vi "nirviRandomDataMultiElementFPGAFIFO.vi"(0 "Method":T1, 1 "Fifo":T2={"displayName"="", "hardwareName"="", "dataType"=enum."I16", "elementTypeDescriptor"=variant, "terminalTypeDescriptor"=variant, "requestedNumberOfElements"=2, "memoryType"=enum."Look-Up Table", "arbitrationForInterfaceA"=enum."Arbitrate if Multiple Requestors Only", "numberOfElementsPerRead"=1, "arbitrationForInterfaceB"=enum."Always Arbitrate", "numberOfElementsPerWrite"=1, "VI_Defined"=FALSE, "type"=enum."Target-Scoped", "initializationParameters"={"initialized"=FALSE, "VI_Path"=path "", "initialData"=variant}, "disableOnOverflow/Underflow"=FALSE, "interfaceConfiguration"=enum."Read A-Write B", "controlLogic"=enum."Slice Fabric", "actualNumberOfElements"=1027, "dramSelection"="", "dramMaxOustandingRequests"=0, "dramIncludeByteEnables"=FALSE, "dramGrantTime"=0, "fullEmulation"=FALSE, "memoryInMultipleClockDomains"=FALSE, "memoryLatency"=1} {"memoryLatency" items=["0", "1", "2", "3"]}, 3 "element in":variant, 5 "error in (no error)":errorcluster, 7 "Element Datatype":i32, 8 "In SCTL":bool, 9 "Input Valid?":bool, 11 "Timeout (ms)":i32, 13 "Ready for Output?":bool) -> (14 "element out":variant, 15 "Timed out":bool, 16 "Ready for Input":bool, 17 "count":u32, 18 "Output Valid":bool, 19 "error out":errorcluster)   [LabVIEW 2020]
uses:
  <vilib>/rvi/DataTransferAndStorage/Container/Common/niFpgaContainerState.ctl
  <vilib>/rvi/DataTransferAndStorage/Container/Common/niFpgaDataTypeControl.ctl
  <vilib>/rvi/DataTransferAndStorage/Container/Common/niFpgaContainerImplementationControl.ctl
  <vilib>/rvi/DataTransferAndStorage/Container/Common/niFpgaContainerArbitrationOptionsControl.ctl
  <vilib>/rvi/DataTransferAndStorage/Container/Common/niFpgaTransferTypeControl.ctl
  <vilib>/rvi/DataTransferAndStorage/Container/Common/niFpgaContainerInitializationParameters.ctl
  <vilib>/rvi/Memory/Memory_Types/niFpgaMemoryInterfaceConfiguration.ctl
  <vilib>/rvi/FIFO/Fifo_Types/niFpgaFifoControlLogicControl.ctl
  <vilib>/rvi/DataTransferAndStorage/Container/Common/niFpgaContainerMemoryLatencyControl.ctl
  <vilib>/rvi/DataTransferAndStorage/Container/Common/niFpgaContainerMethod.ctl
  <vilib>/rvi/interface/RandomDataEmulation/nirviQueueStoreOperation.ctl
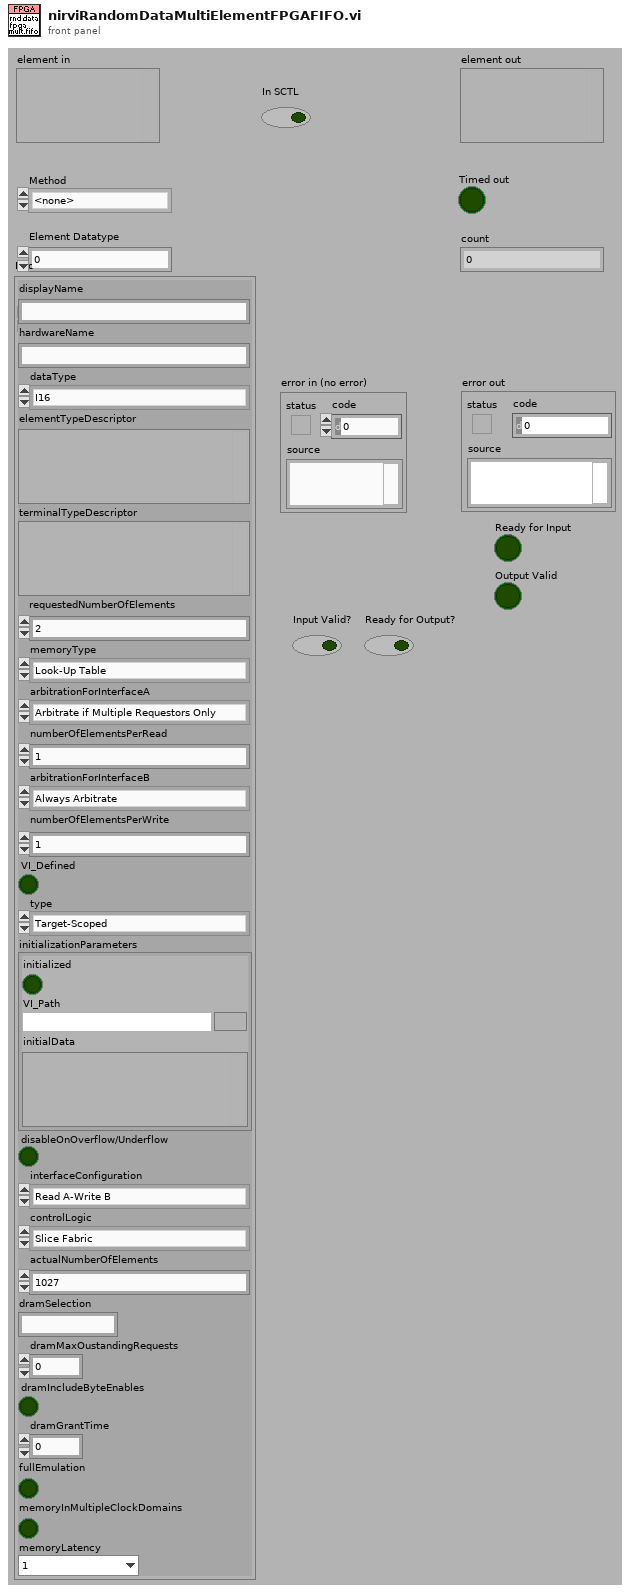
[diagram p1: front panel]
types:
  T1 = typedef "niFpgaContainerMethod.ctl" = enum16{"<none>", "write", "read", "clear", "getNumberOfElementsToWrite", "getNumberOfElementsToRead", "enable", "disable", "flushAndDisable", "getStreamState", "readA", "readB", "dramWrite", "dramWriteWithByteEnables", "dramRequestData", "dramRetrieveData", "readWithoutAcknowledge", "acknowledge", "writeUsingHandshaking", "readUsingHandshaking", "flush"}
  T2 = typedef "niFpgaContainerState.ctl" = cluster{"displayName":string, "hardwareName":string, "dataType":T3, "elementTypeDescriptor":variant, "terminalTypeDescriptor":variant, "requestedNumberOfElements":u32, "memoryType":T4, "arbitrationForInterfaceA":T5, "numberOfElementsPerRead":u32, "arbitrationForInterfaceB":T5, "numberOfElementsPerWrite":u32, "VI_Defined":bool, "type":T6, "initializationParameters":T7, "disableOnOverflow/Underflow":bool, "interfaceConfiguration":T8, "controlLogic":T9, "actualNumberOfElements":u32, "dramSelection":string, "dramMaxOustandingRequests":i32, "dramIncludeByteEnables":bool, "dramGrantTime":u32, "fullEmulation":bool, "memoryInMultipleClockDomains":bool, "memoryLatency":T10}
  T3 = typedef "niFpgaDataTypeControl.ctl" = enum32{"Boolean", "I8", "I16", "I32", "I64", "U8", "U16", "U32", "U64", "FXP", "CustomControl", "SGL"}
  T4 = typedef "niFpgaContainerImplementationControl.ctl" = enum16{"Flip-Flops", "Look-Up Table", "Block Memory", "DRAM", "UltraRAM"}
  T5 = typedef "niFpgaContainerArbitrationOptionsControl.ctl" = enum16{"Always Arbitrate", "Arbitrate if Multiple Requestors Only", "Never Arbitrate"}
  T6 = typedef "niFpgaTransferTypeControl.ctl" = enum16{"Target-Scoped", "Host to Target - DMA", "Target to Host - DMA", "Peer to Peer Reader", "Peer to Peer Writer", "Bidirectional"}
  T7 = typedef "niFpgaContainerInitializationParameters.ctl" = cluster{"initialized":bool, "VI_Path":path, "initialData":variant}
  T8 = typedef "niFpgaMemoryInterfaceConfiguration.ctl" = enum16{"Read A-Write B", "Read A-Read B"}
  T9 = typedef "niFpgaFifoControlLogicControl.ctl" = enum16{"Slice Fabric", "Target Optimal", "Built-in"}
  T10 = typedef "niFpgaContainerMemoryLatencyControl.ctl" = u16
  T11 = typedef "nirviQueueStoreOperation.ctl" = enum16{"Make New Queue", "Get Queue", "Resize Queue", "Close Queues", "Make New Lock", "Get Lock", "Get Host Fifo Size"}
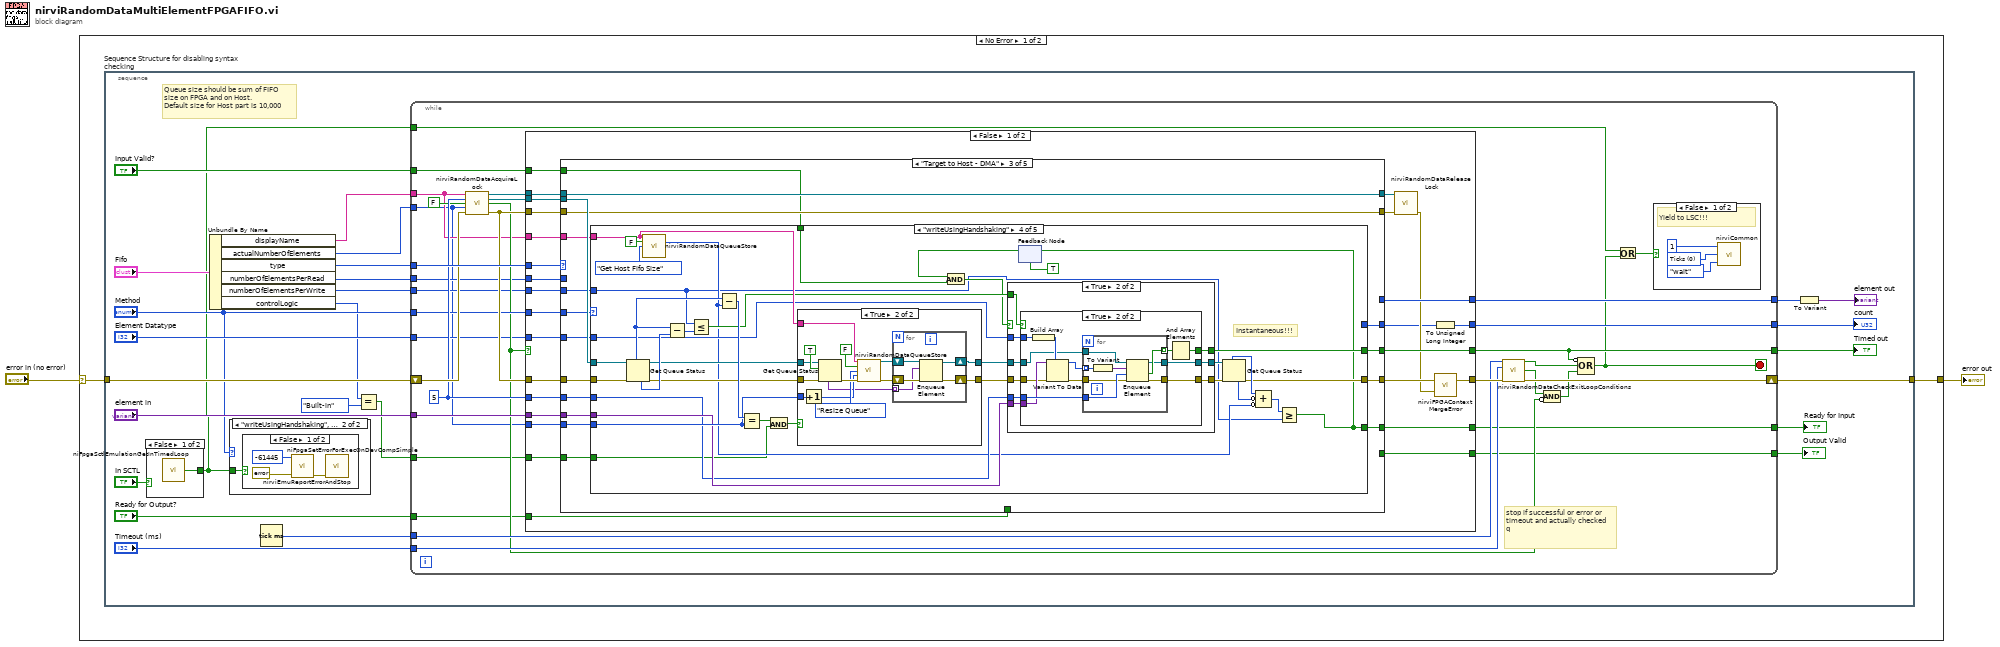
[diagram p0: block diagram]
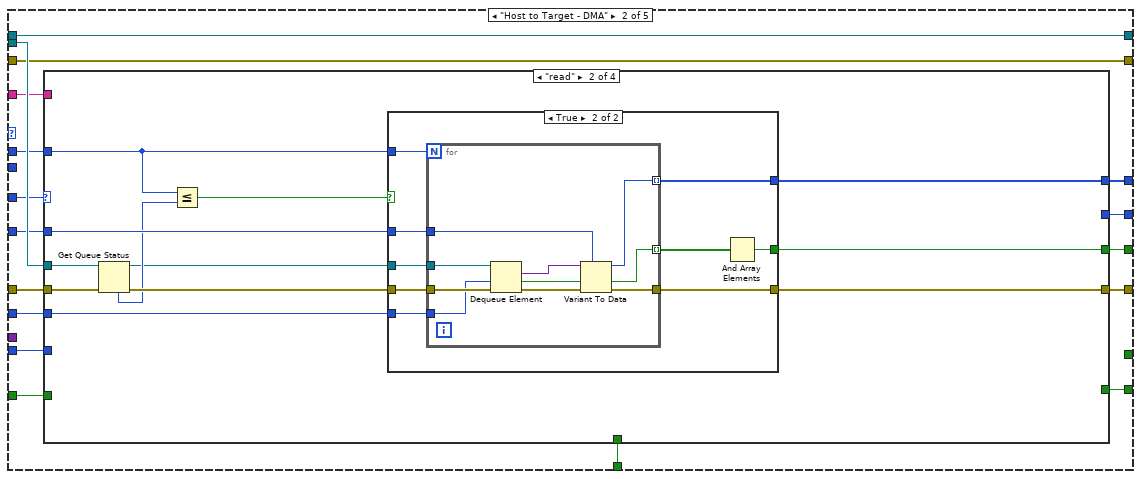
[diagram p7: hidden frame]
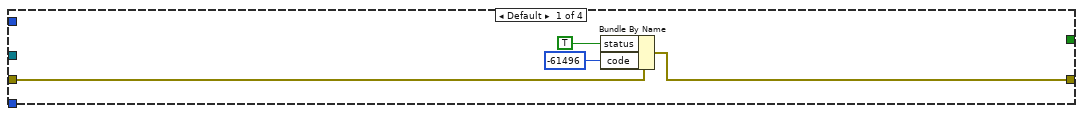
[diagram p8: hidden frame]
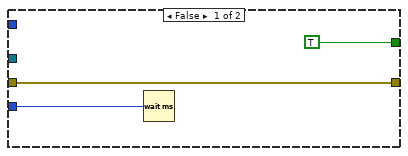
[diagram p9: hidden frame]
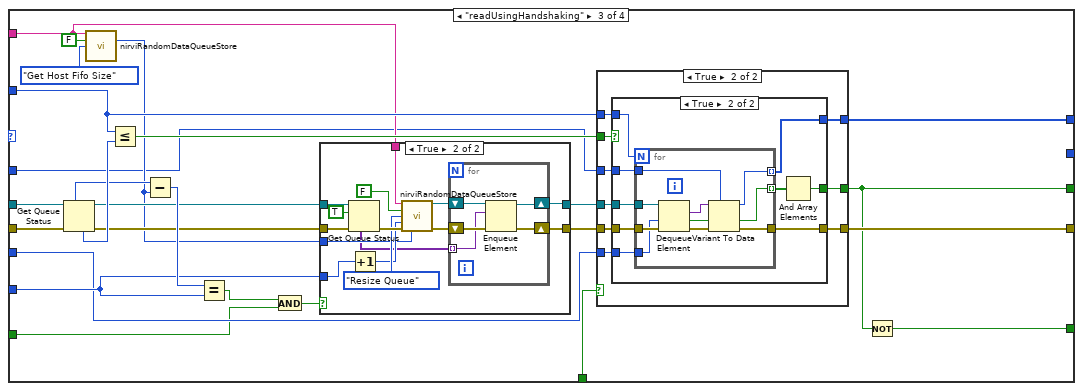
[diagram p10: hidden frame]
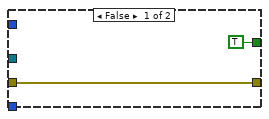
[diagram p11: hidden frame]
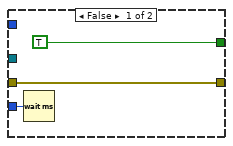
[diagram p12: hidden frame]
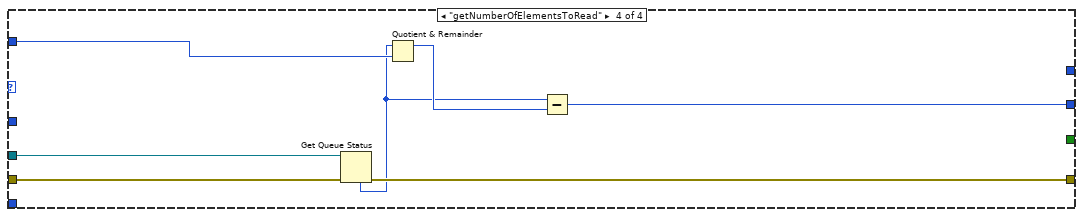
[diagram p14: hidden frame]
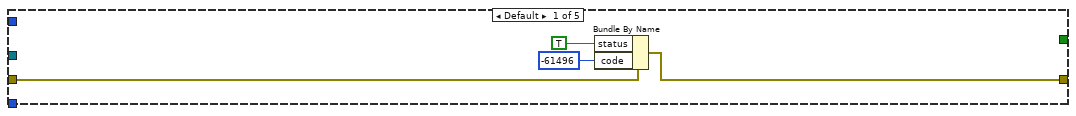
[diagram p15: hidden frame]
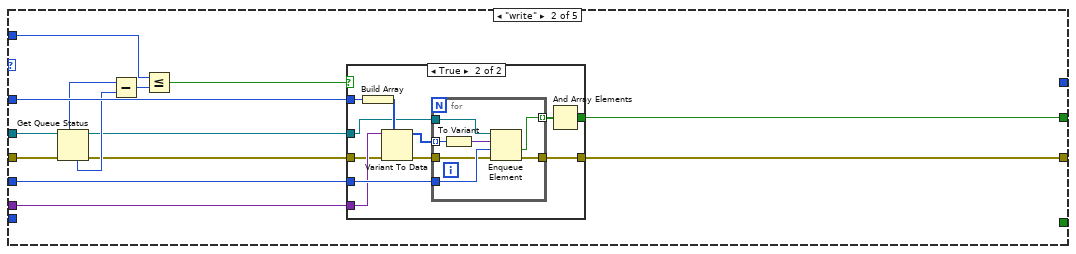
[diagram p16: hidden frame]
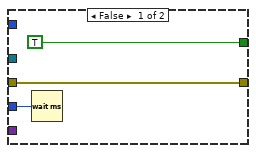
[diagram p17: hidden frame]
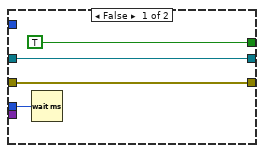
[diagram p20: hidden frame]
diagram:
  n1 = case shown="No Error" "error in (no error)" {
    selector: "error in (no error)" -> [w4 w415]
    tunnel: [w3 w415] -> w2
    frame No Error {
      n2 = stacked-sequence "Sequence Structure for disabling syntax checking" {
        tunnel: w4 -> [w17]
        tunnel: [w29] -> w3
        frame #0 {
          # "Queue size should be sum of FIFO\nsize on FPGA and on Host.\nDefault size for Host part is 10,000"
          n3 = case shown="False" "In SCTL" {
            selector: "In SCTL" -> [_ w32]
            tunnel: [w31 w32] -> w7
            frame False {
              n4 = call <vilib>:"niFpgaSctlEmulationGetInTimedLoop.vi"() -> ("x != 0?"=w31:bool)  [unwired: 15 in]
            }
            frame True {
            }
          }
          n5 = Unbundle By Name("Fifo") -> ("displayName"=w27:string, "actualNumberOfElements"=w25:u32, "type"=w24:T6, "numberOfElementsPerRead"=w20:u32, "numberOfElementsPerWrite"=w19:u32, "controlLogic"=w11:T9)
          n6 = case shown="\"writeUsingHandshaking\", \"readUsingHandshaking\"" "Method" {
            tunnel: w7 -> [_ w33]
            frame Default {
            }
            frame "writeUsingHandshaking", "readUsingHandshaking" {
              n7 = case shown="False" w33 {
                frame False {
                  n8 = call <vilib>:"niFpgaSetErrorForExecOnDevCompSimple.vi"("error code"=-61445, "error in"=errorcluster {"status"=FALSE, "code"=0, "source"=""}) -> ("error out"=w36:errorcluster)  [unwired: 13 in]
                  n9 = call <vilib>:"nirviEmuReportErrorAndStop.vi"("error to report"=w36) -> ()  [unwired: 1 in, 14 out]
                }
                frame True {
                }
              }
            }
          }
          n10 = Tick Count (ms)() -> (millisecond timer value=w28:u32)
          n11 = Equal?(x=w11, y=niFpgaFifoControlLogicControl."Built-in") -> (x = y?=w9:bool)
          n12 = while {
            tunnel: w24 -> [w67]
            tunnel: "element in" -> [w69]
            tunnel: "Timeout (ms)" -> [w63]
            tunnel: [w68] -> w6
            tunnel: [w55] -> w22
            tunnel: w28 -> [w64]
            tunnel: w27 -> [w46]
            shift-right: [w66] -> w29
            shift-left: w17 -> [w62]
            tunnel: w25 -> [w45]
            tunnel: "Method" -> [w56]
            tunnel: [w54] -> w21
            tunnel: "Element Datatype" -> [w49]
            tunnel: w20 -> [w48]
            tunnel: w19 -> [w47]
            tunnel: "Ready for Output?" -> [w44]
            tunnel: [w43] -> w14
            tunnel: "Input Valid?" -> [w42]
            tunnel: [w41] -> w12
            tunnel: w9 -> [w40]
            tunnel: w7 -> [w38]
            stop <- w39 stop-if-true
            w60 = 5 ("ms timeout (-1)")
            # "stop if successful or error or \ntimeout and actually checked q"
            n13 = call <vilib>:"nirviRandomDataAcquireLock.vi"("name"=w46, "ms timeout (-1)"=w60, "Host?"=FALSE, "fpga fifo size"=w45, "error in (no error)"=w62) -> ("lock out"=w61:refnum<queue>, "queue out"=w58:refnum<queue>, "timed out"=w53:bool, "error out"=w57:errorcluster)  [unwired: 7 out]
            n14 = case shown="False" w53 {
              selector: w53 -> [_ w414]
              tunnel: w69 -> [w85 _]
              tunnel: w60 -> [w99 _]
              tunnel: [w98 _] -> w68
              tunnel: [w94 w413] -> w65
              tunnel: [w97 w414] -> w55
              tunnel: w67 -> [w96 _]
              tunnel: w57 -> [w91 w413]
              tunnel: w61 -> [w86 _]
              tunnel: w58 -> [w92 _]
              tunnel: w57 -> [w89 _]
              tunnel: w56 -> [w88 _]
              tunnel: [w83 _] -> w54
              tunnel: w49 -> [w82 _]
              tunnel: w48 -> [w81 _]
              tunnel: w47 -> [w80 _]
              tunnel: w46 -> [w79 _]
              tunnel: w45 -> [w78 _]
              tunnel: w44 -> [w77 _]
              tunnel: [w76 _] -> w43
              tunnel: w42 -> [w75 _]
              tunnel: [w74 _] -> w41
              tunnel: w40 -> [w73 _]
              frame False {
                n15 = case shown="\"Target to Host - DMA\"" w96 {
                  tunnel: w99 -> [_ w118 w259 _ _]
                  tunnel: [_ w117 w257 _ _] -> w97
                  tunnel: [w102 w119 w260 w406 w407] -> w95
                  tunnel: [_ w109 _ _ _] -> w98
                  tunnel: w85 -> [_ _ w258 _ _]
                  tunnel: w91 -> [w102 w116 w256 w406 w408]
                  tunnel: w92 -> [_ w115 w255 _ _]
                  tunnel: [w101 w114 w254 w405 w409] -> w90
                  tunnel: w89 -> [w101 w114 w254 w405 w409]
                  tunnel: w88 -> [_ w112 w252 _ _]
                  tunnel: [w100 w113 w253 w404 w412] -> w87
                  tunnel: w86 -> [w100 w113 w253 w404 w412]
                  tunnel: [_ w111 w244 _ _] -> w84
                  tunnel: w82 -> [_ w110 w251 _ _]
                  tunnel: w81 -> [_ w108 _ _ _]
                  tunnel: w80 -> [_ _ w250 _ _]
                  tunnel: w79 -> [_ w107 w249 _ _]
                  tunnel: w78 -> [_ w106 w248 _ _]
                  tunnel: w77 -> [_ w105 _ _ _]
                  tunnel: [_ w104 _ _ _] -> w76
                  tunnel: w75 -> [_ _ w247 _ _]
                  tunnel: [_ _ w246 _ _] -> w74
                  tunnel: w73 -> [_ w103 w245 _ _]
                  frame "Target-Scoped" {
                    # "Not a DMA FIFO"
                  }
                  frame "Host to Target - DMA" {
                    n16 = case shown="\"read\"" w112 {
                      tunnel: [w120 w135 w182 w243] -> w119
                      tunnel: w118 -> [_ w133 w165 _]
                      tunnel: [_ w132 w162 _] -> w117
                      tunnel: w116 -> [w121 w131 w180 w241]
                      tunnel: w115 -> [_ w127 w177 w242]
                      tunnel: [_ _ _ w237] -> w111
                      tunnel: w110 -> [_ w134 w160 _]
                      tunnel: [_ w124 w181 _] -> w109
                      tunnel: w108 -> [_ w129 w179 w239]
                      tunnel: w107 -> [_ _ w171 _]
                      tunnel: w106 -> [_ _ w167 _]
                      tunnel: w105 -> [_ _ w163 _]
                      tunnel: [_ _ w161 _] -> w104
                      tunnel: w103 -> [_ _ w158 _]
                      frame Default {
                        n17 = Bundle By Name(cluster=w121, "status"=TRUE, "code"=-61496) -> (w120:errorcluster)
                      }
                      frame "read" {
                        n18 = Get Queue Status(queue=w127, error in (no error)=w131) -> (queue out=w126:refnum<queue>, error out=w130:errorcluster, # elements in queue=w128:i32)  [unwired: 1 in, 5 out]
                        n19 = Less Or Equal?(x=w129, y=w128) -> (x <= y?=w125:bool)
                        n20 = case shown="True" w125 {
                          tunnel: [w138 w147] -> w135
                          tunnel: w134 -> [_ w146]
                          tunnel: w133 -> [w136 w145]
                          tunnel: [TRUE ("timed out?") w139] -> w132
                          tunnel: [_ w144] -> w124
                          tunnel: w130 -> [w138 w143]
                          tunnel: w129 -> [_ w142]
                          tunnel: w126 -> [_ w141]
                          frame False {
                            n21 = Wait (ms)(milliseconds to wait=w136) -> ()  [unwired: 1 out]
                          }
                          frame True {
                            n22 = for {
                              N: w142 -> [_]
                              tunnel: [w156] -> w140 mode=indexing
                              tunnel: [w152] -> w147
                              tunnel: [w150] -> w144 mode=indexing
                              tunnel: w143 -> [w155]
                              tunnel: w146 -> [w151]
                              tunnel: w145 -> [w149]
                              tunnel: w141 -> [w148]
                              n23 = Dequeue Element(queue=w148, timeout in ms (-1)=w149, error in (no error)=w155) -> (element=w154:variant, timed out?=w156:bool, error out=w153:errorcluster)  [unwired: 1 out]
                              n24 = Variant To Data(error in=w153, type=w151, Variant=w154) -> (data=w150:i32, error out=w152:errorcluster)
                            }
                            n25 = And Array Elements(Boolean array=w140) -> (logical AND=w139:bool)
                          }
                        }
                      }
                      frame "readUsingHandshaking" {
                        n26 = Get Queue Status(queue=w177, error in (no error)=w180) -> (queue out=w170:refnum<queue>, max queue size=w173:i32, error out=w168:errorcluster, # elements in queue=w178:i32)  [unwired: 1 in, 4 out]
                        n27 = call <vilib>:"nirviRandomDataQueueStore.vi"("queue name"=w171, "Host?"=FALSE, "queue operation"=nirviQueueStoreOperation."Get Host Fifo Size") -> ("host fifo size out"=w166:u32)  [unwired: 9 in, 3 out]
                        n28 = Less Or Equal?(x=w179, y=w178) -> (x <= y?=w176:bool)
                        n29 = Subtract(x=w173, y=w166) -> (x-y=w172:u32)
                        n30 = Equal?(x=w172, y=w167) -> (x = y?=w159:bool)
                        n31 = And(x=w159, y=w158) -> (x .and. y?=w157:bool)
                        n32 = case shown="True" w157 {
                          tunnel: w168 -> [w215 w231]
                          tunnel: w170 -> [w216 w230]
                          tunnel: w171 -> [_ w227]
                          tunnel: w167 -> [_ w224]
                          tunnel: w166 -> [_ w222]
                          tunnel: [w216 w219] -> w169
                          tunnel: [w215 w217] -> w164
                          frame False {
                          }
                          frame True {
                            n33 = Get Queue Status(queue=w230, return elements? (F)=TRUE, error in (no error)=w231) -> (error out=w228:errorcluster, elements=w221:variant[])  [unwired: 6 out]
                            n34 = Increment(x=w224) -> (x+1=w223:u32)
                            n35 = call <vilib>:"nirviRandomDataQueueStore.vi"("queue name"=w227, "Host?"=FALSE, "queue operation"=nirviQueueStoreOperation."Resize Queue", "fpga fifo size"=w223, "error in (no error)"=w228, "host fifo size"=w222) -> ("queue out"=w220:refnum<queue>, "error out"=w218:errorcluster)  [unwired: 6 in, 2 out]
                            n36 = for {
                              tunnel: w221 -> [w234] mode=indexing
                              shift-right: [w232] -> w219
                              shift-left: w220 -> [w235]
                              shift-right: [w233] -> w217
                              shift-left: w218 -> [w236]
                              n37 = Enqueue Element(queue=w235, element=w234, error in (no error)=w236) -> (queue out=w232:refnum<queue>, error out=w233:errorcluster)  [unwired: 1 in, 1 out]
                            }
                          }
                        }
                        n38 = case shown="True" w163 {
                          tunnel: [w184 w193] -> w182
                          tunnel: [TRUE ("timed out?") w192] -> w162
                          tunnel: [_ w191] -> w181
                          tunnel: w179 -> [_ w190]
                          tunnel: w176 -> [_ w189]
                          tunnel: w169 -> [_ w188]
                          tunnel: w165 -> [_ w187]
                          tunnel: w164 -> [w184 w186]
                          tunnel: w160 -> [_ w185]
                          frame False {
                          }
                          frame True {
                            n39 = case shown="True" w189 {
                              tunnel: [w196 w205] -> w193
                              tunnel: w185 -> [_ w204]
                              tunnel: w187 -> [w194 w203]
                              tunnel: [TRUE ("timed out?") w199] -> w192
                              tunnel: [_ w197] -> w191
                              tunnel: w186 -> [w196 w202]
                              tunnel: w190 -> [_ w198]
                              tunnel: w188 -> [_ w201]
                              frame False {
                                n40 = Wait (ms)(milliseconds to wait=w194) -> ()  [unwired: 1 out]
                              }
                              frame True {
                                n41 = for {
                                N: w198 -> [_]
                                tunnel: [w214] -> w200 mode=indexing
                                tunnel: [w210] -> w205
                                tunnel: [w208] -> w197 mode=indexing
                                tunnel: w202 -> [w213]
                                tunnel: w204 -> [w209]
                                tunnel: w203 -> [w207]
                                tunnel: w201 -> [w206]
                                n42 = Dequeue Element(queue=w206, timeout in ms (-1)=w207, error in (no error)=w213) -> (element=w212:variant, timed out?=w214:bool, error out=w211:errorcluster)  [unwired: 1 out]
                                n43 = Variant To Data(error in=w211, type=w209, Variant=w212) -> (data=w208:i32, error out=w210:errorcluster)
                                }
                                n44 = And Array Elements(Boolean array=w200) -> (logical AND=w199:bool)
                              }
                            }
                          }
                        }
                        n45 = Not(x=w162) -> (.not. x?=w161:bool)
                      }
                      frame "getNumberOfElementsToRead" {
                        n46 = Get Queue Status(queue=w242, error in (no error)=w241) -> (error out=w243:errorcluster, # elements in queue=w238:i32)  [unwired: 1 in, 6 out]
                        n47 = Quotient & Remainder(x=w238, y=w239) -> (x-y*floor(x/y)=w240:u32)  [unwired: 1 out]
                        n48 = Subtract(x=w238, y=w240) -> (x-y=w237:u32)
                      }
                    }
                  }
                  frame "Target to Host - DMA" {
                    n49 = case shown="\"writeUsingHandshaking\"" w252 {
                      tunnel: [w261 w278 w300 w307 w401] -> w260
                      tunnel: w259 -> [_ w277 _ w320 _]
                      tunnel: w258 -> [_ w274 _ w321 _]
                      tunnel: [_ w275 _ w335 _] -> w257
                      tunnel: w256 -> [w262 w271 w300 w333 w402]
                      tunnel: w255 -> [_ w269 _ w332 w403]
                      tunnel: w251 -> [_ w276 _ w318 _]
                      tunnel: w250 -> [_ w266 _ w301 _]
                      tunnel: w249 -> [_ _ _ w326 w398]
                      tunnel: w248 -> [_ _ _ w323 _]
                      tunnel: w247 -> [_ _ _ w314 _]
                      tunnel: [_ _ _ w302 _] -> w246
                      tunnel: w245 -> [_ _ _ w304 _]
                      tunnel: [_ _ _ _ w395] -> w244
                      frame Default {
                        n50 = Bundle By Name(cluster=w262, "status"=TRUE, "code"=-61496) -> (w261:errorcluster)
                      }
                      frame "write" {
                        n51 = Get Queue Status(queue=w269, error in (no error)=w271) -> (queue out=w268:refnum<queue>, max queue size=w273:i32, error out=w270:errorcluster, # elements in queue=w272:i32)  [unwired: 1 in, 4 out]
                        n52 = Subtract(x=w273, y=w272) -> (x-y=w267:i32)
                        n53 = Less Or Equal?(x=w266, y=w267) -> (x <= y?=w265:bool)
                        n54 = case shown="True" w265 {
                          tunnel: [w280 w292] -> w278
                          tunnel: w277 -> [w279 w291]
                          tunnel: w276 -> [_ w288]
                          tunnel: [TRUE w285] -> w275
                          tunnel: w274 -> [_ w284]
                          tunnel: w270 -> [w280 w283]
                          tunnel: w268 -> [_ w282]
                          frame False {
                            n55 = Wait (ms)(milliseconds to wait=w279) -> ()  [unwired: 1 out]
                          }
                          frame True {
                            n56 = Build Array(w288) -> (w286:i32[])
                            n57 = Variant To Data(error in=w283, type=w286, Variant=w284) -> (data=w287:i32[], error out=w289:errorcluster)
                            n58 = for {
                              tunnel: [w299] -> w292
                              tunnel: w291 -> [w298]
                              tunnel: [w297] -> w290 mode=indexing
                              tunnel: w282 -> [w296]
                              tunnel: w289 -> [w295]
                              tunnel: w287 -> [w294] mode=indexing
                              n59 = To Variant(anything=w294) -> (Variant=w293:variant)
                              n60 = Enqueue Element(queue=w296, element=w293, timeout in ms (-1)=w298, error in (no error)=w295) -> (timed out?=w297:bool, error out=w299:errorcluster)  [unwired: 1 out]
                            }
                            n61 = And Array Elements(Boolean array=w290) -> (logical AND=w285:bool)
                          }
                        }
                      }
                      frame "flush" {
                      }
                      frame "writeUsingHandshaking" {
                        # "Instantaneous!!!"
                        n62 = Get Queue Status(queue=w332, error in (no error)=w333) -> (queue out=w325:refnum<queue>, max queue size=w328:i32, error out=w324:errorcluster, # elements in queue=w334:i32)  [unwired: 1 in, 4 out]
                        n63 = call <vilib>:"nirviRandomDataQueueStore.vi"("queue name"=w326, "Host?"=FALSE, "queue operation"=nirviQueueStoreOperation."Get Host Fifo Size") -> ("host fifo size out"=w309:u32)  [unwired: 9 in, 3 out]
                        n64 = Subtract(x=w328, y=w334) -> (x-y=w331:i32)
                        n65 = Less Or Equal?(x=w301, y=w331) -> (x <= y?=w316:bool)
                        n66 = Subtract(x=w328, y=w309) -> (x-y=w327:u32)
                        n67 = Equal?(x=w327, y=w323) -> (x = y?=w306:bool)
                        n68 = And(x=w306, y=w304) -> (x .and. y?=w305:bool)
                        n69 = case shown="True" w305 {
                          tunnel: w324 -> [w372 w386]
                          tunnel: [w371 w378] -> w319
                          tunnel: [w372 w376] -> w322
                          tunnel: w325 -> [w371 w375]
                          tunnel: w323 -> [_ w374]
                          tunnel: w326 -> [_ w373]
                          frame False {
                          }
                          frame True {
                            n70 = Increment(x=w374) -> (x+1=w381:u32)
                            n71 = Get Queue Status(queue=w375, return elements? (F)=TRUE, error in (no error)=w386) -> (error out=w384:errorcluster, elements=w380:variant[])  [unwired: 6 out]
                            n72 = call <vilib>:"nirviRandomDataQueueStore.vi"("queue name"=w373, "Host?"=FALSE, "queue operation"=nirviQueueStoreOperation."Resize Queue", "fpga fifo size"=w381, "error in (no error)"=w384) -> ("queue out"=w379:refnum<queue>, "error out"=w377:errorcluster)  [unwired: 7 in, 2 out]
                            n73 = for {
                              tunnel: w380 -> [w389] mode=indexing
                              shift-right: [w387] -> w378
                              shift-left: w379 -> [w390]
                              shift-right: [w388] -> w376
                              shift-left: w377 -> [w391]
                              n74 = Enqueue Element(queue=w390, element=w389, error in (no error)=w391) -> (queue out=w387:refnum<queue>, error out=w388:errorcluster)  [unwired: 1 in, 1 out]
                            }
                          }
                        }
                        n75 = feedback #1(TRUE) -> (w315:bool)
                        n76 = And(x=w315, y=w314) -> (x .and. y?=w308:bool)
                        n77 = case shown="True" w308 {
                          tunnel: [w337 w346] -> w313
                          tunnel: [_ w345] -> w335
                          tunnel: w322 -> [w337 w344]
                          tunnel: w321 -> [_ w343]
                          tunnel: w320 -> [_ w342]
                          tunnel: w319 -> [w336 w341]
                          tunnel: w318 -> [_ w340]
                          tunnel: w316 -> [_ w339]
                          tunnel: [w336 w338] -> w312
                          frame False {
                          }
                          frame True {
                            n78 = case shown="True" w339 {
                              tunnel: [w349 w362] -> w346
                              tunnel: w342 -> [w348 w361]
                              tunnel: w340 -> [_ w358]
                              tunnel: [TRUE w355] -> w345
                              tunnel: w343 -> [_ w354]
                              tunnel: w344 -> [w349 w353]
                              tunnel: w341 -> [w347 w352]
                              tunnel: [w347 w351] -> w338
                              frame False {
                                n79 = Wait (ms)(milliseconds to wait=w348) -> ()  [unwired: 1 out]
                              }
                              frame True {
                                n80 = Build Array(w358) -> (w356:i32[])
                                n81 = Variant To Data(error in=w353, type=w356, Variant=w354) -> (data=w357:i32[], error out=w359:errorcluster)
                                n82 = for {
                                tunnel: [w370] -> w362
                                tunnel: w361 -> [w369]
                                tunnel: [w368] -> w360 mode=indexing
                                tunnel: w352 -> [w367]
                                tunnel: w359 -> [w366]
                                tunnel: w357 -> [w365] mode=indexing
                                tunnel: [w363] -> w351
                                n83 = To Variant(anything=w365) -> (Variant=w364:variant)
                                n84 = Enqueue Element(queue=w367, element=w364, timeout in ms (-1)=w369, error in (no error)=w366) -> (queue out=w363:refnum<queue>, timed out?=w368:bool, error out=w370:errorcluster)
                                }
                                n85 = And Array Elements(Boolean array=w360) -> (logical AND=w355:bool)
                              }
                            }
                          }
                        }
                        n86 = Get Queue Status(queue=w312, error in (no error)=w313) -> (max queue size=w311:i32, error out=w307:errorcluster, # elements in queue=w310:i32)  [unwired: 1 in, 5 out]
                        n87 = Compound Arithmetic op=ADD(w311, invert w310, invert w309) -> (w303:u32)
                        n88 = Greater Or Equal?(x=w303, y=w301) -> (x >= y?=w302:bool)
                        n89 = feedback-in #1(w302) -> ()
                      }
                      frame "getNumberOfElementsToWrite" {
                        n90 = call <vilib>:"nirviRandomDataQueueStore.vi"("queue name"=w398, "Host?"=FALSE, "queue operation"=nirviQueueStoreOperation."Get Host Fifo Size") -> ("host fifo size out"=w394:u32)  [unwired: 9 in, 3 out]
                        n91 = Get Queue Status(queue=w403, error in (no error)=w402) -> (max queue size=w393:i32, error out=w401:errorcluster, # elements in queue=w392:i32)  [unwired: 1 in, 5 out]
                        n92 = Subtract(x=w393, y=w394) -> (x-y=w396:u32)
                        n93 = Subtract(x=w393, y=w392) -> (x-y=w397:i32)
                        n94 = Max & Min(x=w396, y=w397) -> (min(x,y)=w395:u32)  [unwired: 1 out]
                      }
                    }
                  }
                  frame "Peer to Peer Reader", "Peer to Peer Writer" {
                    # "No emulation support"
                  }
                  frame "Bidirectional" {
                    # "Other methods aren't supported by FIFOs."
                    n95 = Bundle By Name(cluster=w408, "status"=TRUE, "code"=-61496) -> (w407:errorcluster)
                  }
                }
                n96 = call <vilib>:"nirviRandomDataReleaseLock.vi"("lock in"=w87, "error in (no error)"=w90) -> ("error out"=w93:errorcluster)  [unwired: 13 out]
                n97 = To Unsigned Long Integer(number=w84) -> (unsigned 32bit integer=w83:u32)
                n98 = call <vilib>:"nirviFPGAContextMergeError.vi"("error 2"=w93, "error 1"=w95) -> ("error out"=w94:errorcluster)
              }
              frame True {
              }
            }
            n99 = call <vilib>:"nirviRandomDataCheckExitLoopConditions.vi"("Start Time"=w64, "Timeout (ms)"=w63, "error in (no error)"=w65) -> ("Error Occurred"=w50:bool, "Timed Out"=w52:bool, "error out"=w66:errorcluster)  [unwired: 10 out]
            n100 = Compound Arithmetic op=AND(w52, invert w53) -> (w51:bool)
            n101 = Compound Arithmetic op=OR(invert w55, w50, w51) -> (w39:bool)
            n102 = Or(x=w38, y=w39) -> (x .or. y?=w37:bool)
            n103 = case shown="False" w37 {
              frame False {
                w71 = u16 0 items=["Ticks", "µSec", "mSec"] ("Counter Units")
                # "Yield to LSC!!!"
                n104 = call <vilib>:"nirviCommon.vi"("Action"=enum16{"wait", "wait multiple", "tick count"}."wait", "Counter Units"=w71, "Count(uSec)"=u32 1) -> ()  [unwired: 1 out]
              }
              frame True {
              }
            }
          }
          "Timed out" <- w22
          "count" <- w21
          "Ready for Input" <- w12
          "Output Valid" <- w14
          n105 = To Variant(anything=w6) -> (Variant=→"element out":variant)
        }
      }
    }
    frame Error {
    }
  }
  "error out" <- w2
